vi "comm write and receive echo.vi"(8 "error in (no error)":errorcluster, 9 "stop if not equal? (F)":bool, 10 "string to write":string, 11 "Comm Handle":u32) -> (0 "error out":errorcluster, 1 "bytes received":u32, 2 "string received":string, 3 "dup Comm Handle":u32, 5 "bytes written":u32)   [LabVIEW 2017, in "lvserial.lvlib"]
doc: "Writes data to the serial port and received the echo. Note, that this function does not handle the specified termination conditions. It transmits the start end end of transmission string, but it does not return the received echo of these strings."
uses:
  lvserial.lvlib
  lvserial.dll
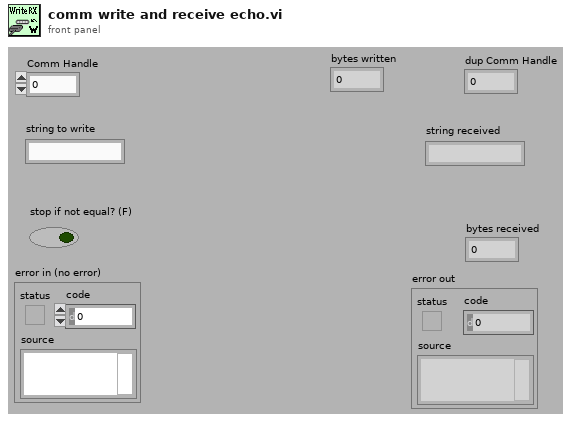
[diagram p1: front panel]
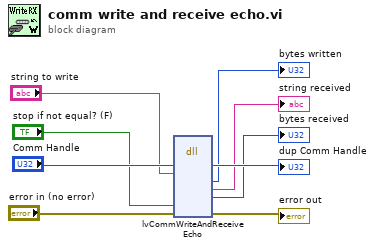
[diagram p0: block diagram]
diagram:
  n1 = dll-call lib="lvserial.dll" fn="lvCommWriteAndReceiveEcho"("hComm"="Comm Handle", "Buffer"="string to write", "stop if not equal? (F)"="stop if not equal? (F)", "error in (no error)"="error in (no error)") -> ("hComm"=→"dup Comm Handle":u32, "pulBytesWritten"=→"bytes written":u32, "shReadBuffer"=→"string received":string, "pulBytesRead"=→"bytes received":u32, "error in (no error)"=→"error out":errorcluster)  [unwired: 6 in, 5 out]
